vi "regSubEvents.vi"(8 "error in (no error)":errorcluster, 11 "SALCommunicator in":refnum<class "SALCommunicatorDL.lvclass">) -> (0 "error out":errorcluster, 2 "SAL Evnts":refnum<event-registration>, 3 "SALCommunicator out":refnum<class "SALCommunicatorDL.lvclass">)   [LabVIEW 2016, in "SALCommunicatorView.lvclass"]
uses:
  SALCommunicatorView.lvclass
  SALCommunicatorDL/SALCommunicatorDL.lvclass
  ts_sallv_exa/SALLV_EXA.lvlib
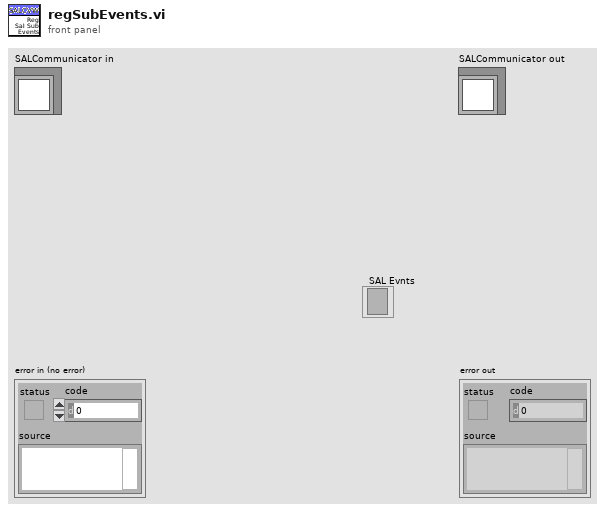
[diagram p1: front panel]
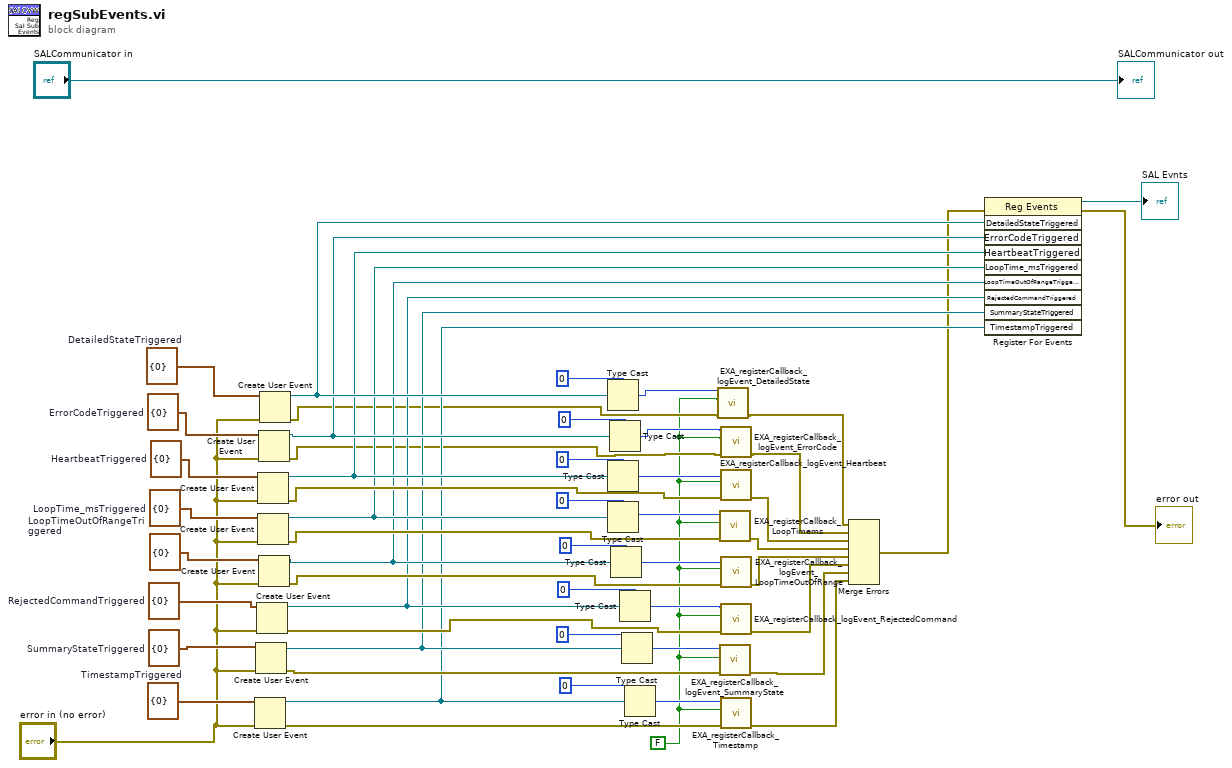
[diagram p0: block diagram]
diagram:
  w26 = cluster{"Data":i32} {"Data"=0}  # ErrorCodeTriggered
  w32 = cluster{"Data":i32} {"Data"=0}  # TimestampTriggered
  w31 = cluster{"Data":i32} {"Data"=0}  # SummaryStateTriggered
  w30 = cluster{"Data":i32} {"Data"=0}  # RejectedCommandTriggered
  w29 = cluster{"Data":i32} {"Data"=0}  # LoopTimeOutOfRangeTriggered
  w28 = cluster{"Data":i32} {"Data"=0}  # LoopTime_msTriggered
  w27 = cluster{"Data":i32} {"Data"=0}  # HeartbeatTriggered
  w33 = cluster{"Data":i32} {"Data"=0}  # DetailedStateTriggered
  w2 = FALSE ("skipOld")
  n1 = Create User Event(user event datatype=w32, error in="error in (no error)") -> (user event=w11:refnum<user-event>, error out=w20:errorcluster)
  n2 = Create User Event(user event datatype=w31, error in="error in (no error)") -> (user event=w12:refnum<user-event>, error out=w21:errorcluster)
  n3 = Create User Event(user event datatype=w30, error in="error in (no error)") -> (user event=w13:refnum<user-event>, error out=w22:errorcluster)
  n4 = Create User Event(user event datatype=w27, error in="error in (no error)") -> (user event=w16:refnum<user-event>, error out=w25:errorcluster)
  n5 = Create User Event(user event datatype=w28, error in="error in (no error)") -> (user event=w15:refnum<user-event>, error out=w24:errorcluster)
  n6 = Create User Event(user event datatype=w26, error in="error in (no error)") -> (user event=w17:refnum<user-event>, error out=w6:errorcluster)
  n7 = Create User Event(user event datatype=w29, error in="error in (no error)") -> (user event=w14:refnum<user-event>, error out=w23:errorcluster)
  n8 = Create User Event(user event datatype=w33, error in="error in (no error)") -> (user event=w18:refnum<user-event>, error out=w3:errorcluster)
  n9 = Type Cast(type=0, x=w18) -> (*(type *) &x=w1:i32)
  n10 = Type Cast(type=0, x=w16) -> (*(type *) &x=w38:i32)
  n11 = Type Cast(type=0, x=w15) -> (*(type *) &x=w39:i32)
  n12 = Type Cast(type=0, x=w17) -> (*(type *) &x=w7:i32)
  n13 = Type Cast(type=0, x=w14) -> (*(type *) &x=w40:i32)
  n14 = Type Cast(type=0, x=w13) -> (*(type *) &x=w45:i32)
  n15 = Type Cast(type=0, x=w12) -> (*(type *) &x=w46:i32)
  n16 = Type Cast(type=0, x=w11) -> (*(type *) &x=w48:i32)
  n17 = call "EXA_registerCallback_logEvent_DetailedState.vi"("error in (no error)"=w3, "skipOld"=w2, "handle"=w1) -> ("error out"=w4:errorcluster)  [unwired: 7 in, 1 out]
  n18 = call "EXA_registerCallback_LoopTimems.vi"("error in (no error)"=w24, "skipOld"=w2, "handle"=w39) -> ("error out"=w35:errorcluster)  [unwired: 7 in, 1 out]
  n19 = call "EXA_registerCallback_logEvent_SummaryState.vi"("error in (no error)"=w21, "skipOld"=w2, "handle"=w46) -> ("error out"=w47:errorcluster)  [unwired: 7 in, 1 out]
  n20 = call "EXA_registerCallback_logEvent_ErrorCode.vi"("error in (no error)"=w6, "skipOld"=w2, "handle"=w7) -> ("error out"=w5:errorcluster)  [unwired: 7 in, 1 out]
  n21 = call "EXA_registerCallback_logEvent_Heartbeat.vi"("error in (no error)"=w25, "skipOld"=w2, "handle"=w38) -> ("error out"=w34:errorcluster)  [unwired: 7 in, 1 out]
  n22 = call "EXA_registerCallback_logEvent_LoopTimeOutOfRange.vi"("error in (no error)"=w23, "skipOld"=w2, "handle"=w40) -> ("error out"=w36:errorcluster)  [unwired: 7 in, 1 out]
  n23 = call "EXA_registerCallback_logEvent_RejectedCommand.vi"("error in (no error)"=w22, "skipOld"=w2, "handle"=w45) -> ("error out"=w37:errorcluster)  [unwired: 7 in, 1 out]
  n24 = call "EXA_registerCallback_Timestamp.vi"("error in (no error)"=w20, "skipOld"=w2, "handle"=w48) -> ("error out"=w49:errorcluster)  [unwired: 7 in, 1 out]
  n25 = Merge Errors(w4, w5, w34, w35, w36, w37, w47, w49) -> (w10:errorcluster)
  n26 = register-events(error in=w10, w18, w17, w16, w15, w14, w13, w12, w11) -> (reference out=→"SAL Evnts":refnum<event-registration>, error out=→"error out":errorcluster)  [unwired: 1 in]
  "SALCommunicator out" <- "SALCommunicator in"
